vi "ILAB_GetVI.vi"(4 "path":string) -> (0 "errorOut":string, 1 "viReference":refnum<vi>)   [LabVIEW 2009]
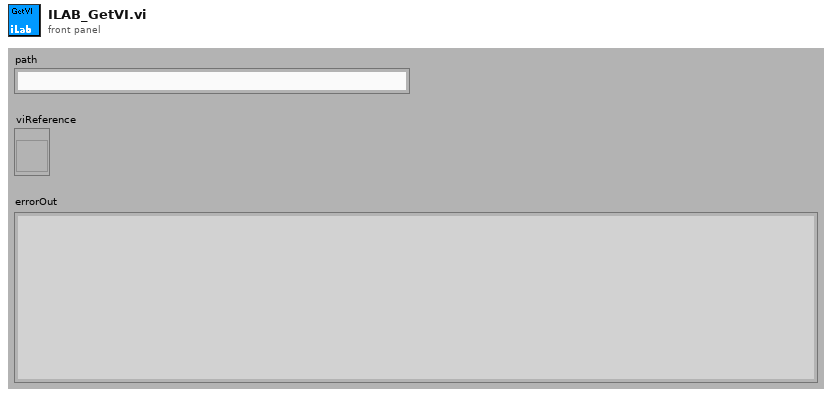
[diagram p1: front panel]
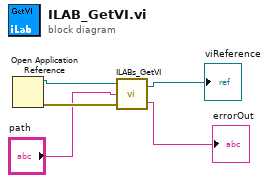
[diagram p0: block diagram]
diagram:
  n1 = Open Application Reference() -> (0:w4:errorcluster, 3:w5:refnum<vi>)  [unwired: 1 in, 3 out]
  n2 = call "ILABs_GetVI.vi"("errorIn"=w4, "path"="path", "appReference"=w5) -> ("errorOut"=→"errorOut":string, "vi reference"=→"viReference":refnum<vi>)
